vi "DDC (Single Channel).vi"(0 "data in":T3, 1 "reset":bool, 5 "start trigger":bool, 9 "enabled":bool, 11 "DDC Parameters":T1={"output sample rate"=1.0, "delay"=0.0, "frequency shift"=0.0, "impairments"={"inline gain I"=0.9999923706054688, "inline gain Q"=0.9999923706054688, "cross gain I"=0.0, "cross gain Q"=0.0, "pre-gain offset I"=0.0, "pre-gain offset Q"=0.0, "post-gain offset I"=0.0, "post-gain offset Q"=0.0}, "phase"=0.0} {"frequency shift" format="%#.48g"}) -> (4 "data out":u32, 6 "number of overflows":u64, 10 "output valid":bool, 14 "dsp reset done":bool)   [LabVIEW 2015]
doc: "Digital downconverter (DDC) for a single channel. Implemented with FPGA-based DSP."
uses:
  <instrlib>/_niInstr/DSP/v1/Shared/Public/IQ Data.ctl
  DDC Parameters.ctl
  <instrlib>/_niInstr/DSP/v1/Shared/Public/IQ Impairments.ctl
  <instrlib>/_niInstr/Basic Elements/v1/FPGA/Private/Count Up U64.vi
  <instrlib>/_niInstr/DSP/v1/FPGA/Public/Sub VIs/IQ Impairments/IQ Impairments - 1 spc.vi
  <instrlib>/_niInstr/DSP/v1/FPGA/Public/Sub VIs/Frequency Shift/Frequency Shift - 1 spc.vi
  <instrlib>/_niInstr/Basic Elements/v1/FPGA/niInstr Basic Elements v1 FPGA.lvlib
  <instrlib>/_niInstr/DSP/v1/FPGA/niInstr DSP v1 FPGA.lvlib
  <instrlib>/niUsrpRio/DSP/v1/FPGA/niUsrpRio DSP v1 FPGA.lvlib
  <instrlib>/_niInstr/DSP/v1/Shared/niInstr DSP v1 Shared.lvlib
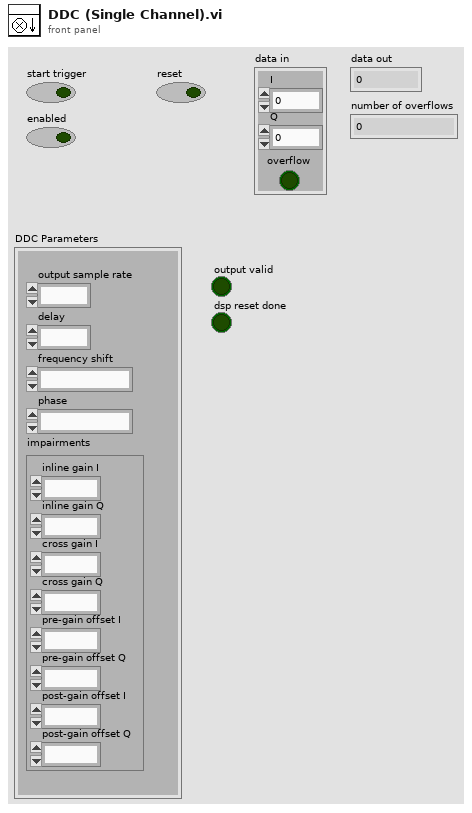
[diagram p1: front panel]
types:
  T1 = typedef "DDC Parameters.ctl" = cluster{"output sample rate":fxp<+,48,1>, "delay":fxp<+/-,16,0>, "frequency shift":fxp<+/-,48,0>, "impairments":T2, "phase":fxp<+/-,21,0>}
  T2 = typedef "niInstr DSP v1 Shared.lvlib/IQ Impairments.ctl" = cluster{"inline gain I":fxp<+/-,18,1>, "inline gain Q":fxp<+/-,18,1>, "cross gain I":fxp<+/-,18,1>, "cross gain Q":fxp<+/-,18,1>, "pre-gain offset I":fxp<+/-,18,1>, "pre-gain offset Q":fxp<+/-,18,1>, "post-gain offset I":fxp<+/-,18,1>, "post-gain offset Q":fxp<+/-,18,1>}
  T3 = typedef "niInstr DSP v1 Shared.lvlib/IQ Data.ctl" = cluster{"I":fxp<+/-,18,1>, "Q":fxp<+/-,18,1>, "overflow":bool}
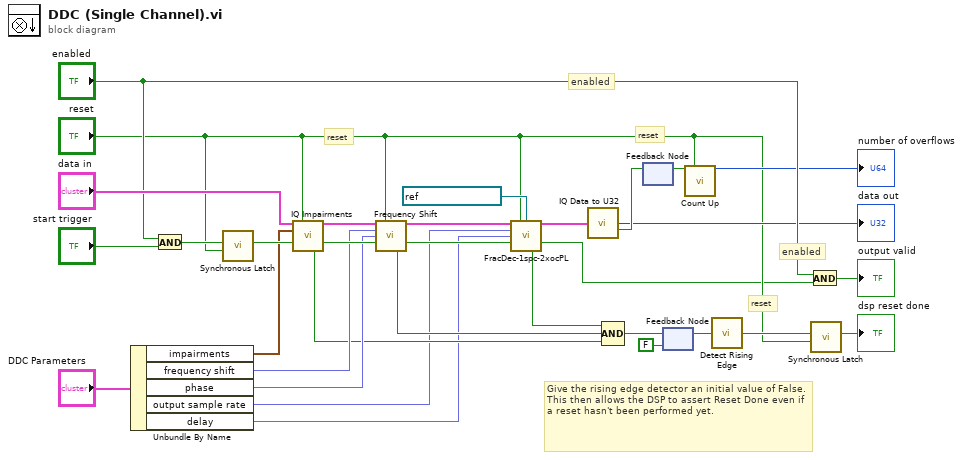
[diagram p0: block diagram]
diagram:
  # "Give the rising edge detector an initial value of False.  This then allows the DSP to assert Reset Done even if a reset hasn't been performed yet."
  # "reset"
  # "reset"
  # "reset"
  # "enabled"
  # "enabled"
  n1 = Unbundle By Name("DDC Parameters") -> ("impairments"=w28:T2, "frequency shift"=w27:fxp<+/-,48,0>, "phase"=w26:fxp<+/-,21,0>, "output sample rate"=w1:fxp<+,48,1>, "delay"=w2:fxp<+/-,16,0>)
  n2 = And(x="enabled", y="start trigger") -> (x .and. y?=w23:bool)
  n3 = call <instrlib>:"Synchronous Latch.vi"("clear"="reset", "set"=w23) -> ("out"=w31:bool)  [unwired: 9 in]
  n4 = call-poly <instrlib>:"IQ Impairments.vi"("data in"="data in", "reset"="reset", "impairments"=w28, "input valid"=w31) -> ("data out"=w32:T3, "output valid"=w30:bool, "ready for input"=w10:bool)  [unwired: 9 in]
  n5 = call-poly <instrlib>:"Frequency Shift.vi"("data in"=w32, "reset"="reset", "frequency shift"=w27, "phase"=w26, "input valid"=w30) -> ("data out"=w7:T3, "output valid"=w3:bool, "ready for input"=w11:bool)  [unwired: 8 in]
  n6 = call <instrlib>:"FracDec-1spc-2xocPL.vi"("data in"=w7, "reset"="reset", "clock x 2"=refnum<k21> "Data Clock x2" ("oversample clock"), "output sample rate"=w1, "delay"=w2, "input valid"=w3) -> ("data out"=w6:T3, "output valid"=w5:bool, "ready for input"=w4:bool)  [unwired: 7 in]
  n7 = call <instrlib>:"IQ Data to U32.vi"("IQ data"=w6) -> ("U32 data"=→"data out":u32, "overflow"=w19:bool)  [unwired: 13 in]
  n8 = Compound Arithmetic op=AND(w4, w11, w10) -> (w12:bool)
  n9 = feedback #1() -> (w18:bool)  [unwired: 1 in]
  n10 = feedback-in #1(w19) -> ()
  n11 = feedback-in #2(w12) -> ()
  n12 = feedback #2(FALSE ("ready for input")) -> (w14:bool)
  n13 = call-poly <instrlib>:"Count Up.vi"("increment"=w18, "reset"="reset") -> ("count out"=→"number of overflows":u64)  [unwired: 13 in]
  n14 = call <instrlib>:"Detect Rising Edge.vi"("signal"=w14) -> ("edge detected"=w29:bool)  [unwired: 14 in]
  n15 = And(x="enabled", y=w5) -> (x .and. y?=→"output valid":bool)
  n16 = call <instrlib>:"Synchronous Latch.vi"("clear"="reset", "set"=w29) -> ("out"=→"dsp reset done":bool)  [unwired: 9 in]
